vi "PH_Beckhoff_PP_Control.constructor.vi"(0 "name":string, 2 "data in":string, 5 "error in(no error)":errorcluster) -> (14 "i ref out":refnum<vi>, 16 "data out":string, 19 "error out":errorcluster)   [LabVIEW 2014, in "PH_Beckhoff_PP_Control.lvlib"]
doc: "This is the constructor of a class.\n\nLicense Agreement for this software:\n\nCopyright (C)\nGesellschaft für Schwerionenforschung, GSI\nPlanckstr. 1\n64291 Darmstadt\nGermany\n\nContact: D.Beck@gsi.de \n\nThis program is free software; you can redistribute it and/or modify it under the terms of the \nGNU General Public License as published by the Free Software Foundation; either version 2 of \nthe license, or (at your option) any later version.\n\nThis program is distributed in the hope that it will be useful, but WITHOUT ANY WARRANTY; \nwithout even the implied warranty of MERCHANTABILITY or FITNESS FOR A PARTICULAR PURPOSE. See the GNU General License for more details (http://www.gnu.org).\n\nGesellschaft für Schwerionenforschung, GSI\nPlanckstr. 1, 64291 Darmstadt, Germany\nFor all questions and ideas contact: M.Richter@gsi.de, H.Brand@gsi.de or D.Beck@gsi.de.\nLast update: 16-JUN-2004"
uses:
  PH_Beckhoff_PP_Control.lvlib
  PH_Basics/PH_PSDBWriter/PH_PSDBWriter.Thread Commands.ctl
  CS_Core/CSSystem/CSSystemLib/CSSystemLib.lvlib
  PH_Beckhoff/PH_Beckhoff.lvlib
  PH_Basics/PH_PSDBWriter/PH_PSDBWriter.lvlib
  PH_Basics/PH_Class/PH_Class.lvlib
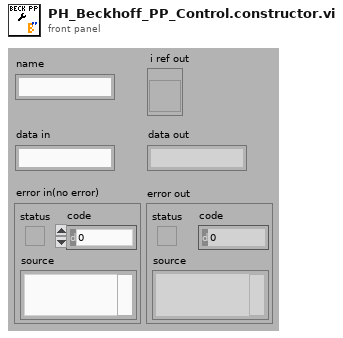
[diagram p1: front panel]
types:
  T1 = enum16{"SetAttribute", "GetAttribute", "CreateAttribute", "DestroyAttribute", "DestroyAllAtributes"}
  T2 = typedef "PH_PSDBWriter.lvlib/PH_PSDBWriter.Thread Commands.ctl" = u16
  T3 = typedef "PH_Beckhoff.lvlib/PH_Beckhoff.constructor Data in.ctl" = cluster{"Default Values":T4, "Description":string, "Hardware configured?":bool, "Activate Change Manager?":bool, "Difference to handle an analog input as change":u32}
  T4 = typedef "PH_Beckhoff.lvlib/PH_Beckhoff.Values.ctl" = cluster{"Sonderklemmen Inputs":T5, "Analog Inputs":T6, "Analog Outputs":T8, "Digital Inputs":T9, "Digital Outputs":T10}
  T5 = typedef "PH_Beckhoff.lvlib/PH_Beckhoff.Sonderklemmen Inputs.ctl" = cluster{"Total Length":u32, "Name":string, "Value":u64, "Quality":bool, "Service ID":i32, "Offset":u32, "Length":u32}[]
  T6 = typedef "PH_Beckhoff.lvlib/PH_Beckhoff.Analog Inputs.ctl" = cluster{"Name":string, "Value":u32, "Quality":bool, "Service ID":i32, "Sca Type":T7}[]
  T7 = typedef "PH_Beckhoff.lvlib/PH_Beckhoff.Scaling Type.ctl" = enum16{"none", "0 ... 15 Bit -> 0 ... 5", "0 ... 15 Bit -> 0 ... 10", "0 ... 15 Bit -> 0 ... 25", "0 ... 15 Bit -> 4 ... 20", "0 ... 15 Bit -> 0 ... 1", "0 ... 15 Bit -> 0 ... 20000", "0 ... 15 Bit -> 0 ... 24000"}
  T8 = typedef "PH_Beckhoff.lvlib/PH_Beckhoff.Analog Outputs.ctl" = cluster{"Name":string, "Value":u32, "Quality":bool, "Wanted Value":u32, "Service ID":i32, "Sca Type":T7}[]
  T9 = typedef "PH_Beckhoff.lvlib/PH_Beckhoff.Digital Inputs.ctl" = cluster{"Name":string, "Value":bool, "Quality":bool, "Service ID":i32, "inverted?":bool}[]
  T10 = typedef "PH_Beckhoff.lvlib/PH_Beckhoff.Digital Outputs.ctl" = cluster{"Name":string, "Value":bool, "Quality":bool, "Wanted Value":bool, "Service ID":i32, "inverted?":bool}[]
  T11 = typedef "PH_Beckhoff_PP_Control.lvlib/PH_Beckhoff_PP_Control.i attribute.ctl" = cluster{"PP Conductivity Control":cluster{"PSDB":cluster{"Status Service ID":i32, "Instance ID":i32, "Data Status":T12, "Ref Status":refnum<vi>, "Error Code":i32}, "Status":cluster{"GUI Ref":refnum<vi>, "Status Service ID":i32, "Status":T13}, "DIs":cluster{"Device on":cluster{"GUI Ref":refnum<vi>, "# in Data":i32}, "Conductivity ok":cluster{"GUI Ref":refnum<vi>, "# in Data":i32}, "Temperature ok":cluster{"GUI Ref":refnum<vi>, "# in Data":i32}, "Alarm":cluster{"GUI Ref":refnum<vi>, "# in Data":i32}}, "PSDB Thread":cluster{"Ref":refnum<vi>, "Q-Ref":refnum<queue>}}, "PP Mercury Control":cluster{"PSDB":cluster{"Status Service ID":i32, "Instance ID":i32, "Data Status":T12, "Ref Status":refnum<vi>, "Error Code":i32}, "Status":cluster{"GUI Ref":refnum<vi>, "Status Service ID":i32, "Status":T13}, "on since:":cluster{"GUI Ref":refnum<vi>, "Service ID":i32, "Time":string}, "DIs":cluster{"Device on":cluster{"GUI Ref":refnum<vi>, "# in Data":i32}, "Alarm":cluster{"GUI Ref":refnum<vi>, "# in Data":i32}}, "AIs":cluster{"Concentration":cluster{"GUI Ref":refnum<vi>, "# in Data":i32}}, "PSDB Thread":cluster{"Ref":refnum<vi>, "Q-Ref":refnum<queue>}}, "PSDB":cluster{"Shot #":i32, "Subsystem":T14}, "PSDB Credentials":T15}
  T12 = typedef "PH_PSDBWriter.lvlib/PH_PSDBWriter.Data Status.ctl" = i16
  T13 = typedef "PH_StatusHandler.lvlib/PH_StatusHandler.Status.ctl" = i16
  T14 = typedef "PH_PSDBWriter.lvlib/PH_PSDBWriter.PHELIX-Subsystems.ctl" = i32
  T15 = typedef "PH_Common.lvlib/PH_Connection.PSDB Credentials.ctl" = cluster{"PW":string, "ID":string, "DS":string}
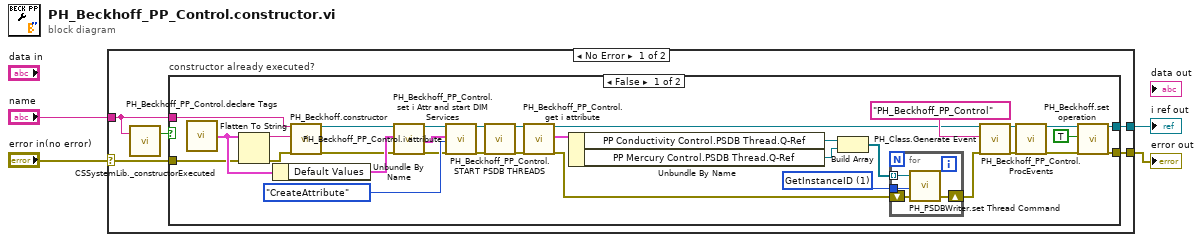
[diagram p0: block diagram]
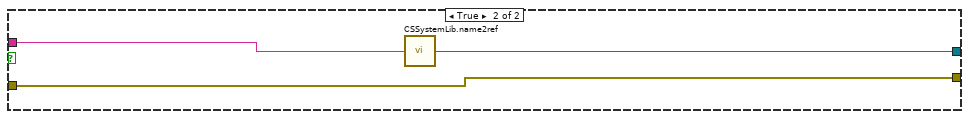
[diagram p2: hidden frame]
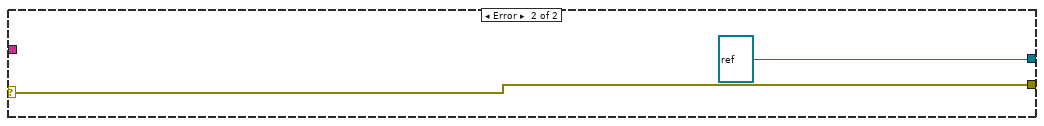
[diagram p3: hidden frame]
diagram:
  n1 = case shown="No Error" "error in(no error)" {
    selector: "error in(no error)" -> [w7 w50]
    tunnel: "name" -> [w6 _]
    tunnel: [w9 refnum<vi> refnum ("obj refnum")] -> w3
    tunnel: [w8 w50] -> w2
    frame No Error {
      n2 = call "CSSystemLib._constructorExecuted.vi"("name"=w6) -> ("constructor executed?"=w5:bool)  [unwired: 18 in]
      n3 = case "constructor already executed?" shown="False" w5 {
        tunnel: [w38 w47] -> w9
        tunnel: [w37 w46] -> w8
        tunnel: w7 -> [w10 w46]
        tunnel: w6 -> [w41 w48]
        frame False {
          w34 = T2 1 items=["None", "GetInstanceID", "WriteToPSDB"] ("PSDB Thread Command")
          n4 = call "PH_Beckhoff_PP_Control.declare Tags.vi"() -> ("Data in cluster"=w28:T3)  [unwired: 1 in]
          n5 = Flatten To String(anything=w28, error in (no error)=w10) -> (data string=w39:string, error out=w40:errorcluster)  [unwired: 2 in, 1 out]
          n6 = Unbundle By Name(w28) -> ("Default Values"=w29:T4)
          n7 = call "PH_Beckhoff.constructor.vi"("name"=w41, "data in"=w39, "error in(no error)"=w40) -> ("i ref out"=w18:refnum<vi>, "error out"=w19:errorcluster)  [unwired: 14 in, 1 out]
          n8 = call "PH_Beckhoff_PP_Control.set i Attr and start DIM Services.vi"("i ref in"=w18, "Values"=w29, "error in"=w19) -> ("i ref out"=w27:refnum<vi>, "i Attr"=w25:T11, "error out"=w26:errorcluster)  [unwired: 14 in]
          n9 = call "PH_Beckhoff_PP_Control.i attribute.vi"("VI Refnum"=w27, "CLASS.i attribute"=w25, "Action"=T1."CreateAttribute", "error in (no error)"=w26) -> ("VI Refnum out"=w23:refnum<vi>, "error out"=w24:errorcluster)  [unwired: 13 in, 1 out]
          n10 = call "PH_Beckhoff_PP_Control.START PSDB THREADS.vi"("VI in"=w23, "error in (no error)"=w24) -> ("VI out"=w22:refnum<vi>, "error out"=w21:errorcluster)  [unwired: 16 in]
          n11 = call "PH_Beckhoff_PP_Control.get i attribute.vi"("i ref in"=w22, "error in (no error)"=w21) -> ("i ref out"=w12:refnum<vi>, "i attribute"=w33:T11, "error out"=w35:errorcluster)  [unwired: 15 in]
          n12 = Unbundle By Name(w33) -> ("PP Conductivity Control.PSDB Thread.Q-Ref"=w32:refnum<queue>, "PP Mercury Control.PSDB Thread.Q-Ref"=w30:refnum<queue>)
          n13 = Build Array(w32, w30) -> (w31:refnum<queue>[])
          n14 = for {
            shift-right: [w44] -> w14
            shift-left: w35 -> [w45]
            tunnel: w34 -> [w43]
            tunnel: w31 -> [w42] mode=indexing
            n15 = call "PH_PSDBWriter.set Thread Command.vi"("error in (no error)"=w45, "PSDB Thread Command"=w43, "Queue in"=w42) -> ("error out"=w44:errorcluster)  [unwired: 2 in]
          }
          n16 = call "PH_Class.Generate Event.vi"("i ref in"=w12, "Class"="PH_Beckhoff_PP_Control", "error in (no error)"=w14) -> ("i ref out"=w11:refnum<vi>, "error out"=w13:errorcluster)  [unwired: 15 in]
          n17 = call "PH_Beckhoff_PP_Control.ProcEvents.vi"("i ref in"=w11, "error in"=w13) -> ("i ref out"=w15:refnum<vi>, "error out"=w16:errorcluster)  [unwired: 16 in]
          n18 = call "PH_Beckhoff.set operation.vi"("VI in"=w15, "operation?"=TRUE, "error in (no error)"=w16) -> ("VI out"=w38:refnum<vi>, "error out"=w37:errorcluster)  [unwired: 15 in]
        }
        frame True {
          n19 = call "CSSystemLib.name2ref.vi"("name"=w48) -> ("obj refnum"=w47:refnum<vi>)
        }
      }
    }
    frame Error {
    }
  }
  "i ref out" <- w3
  "error out" <- w2
